vi "Apply Velocity to Wheels.vi"   [LabVIEW 2017, in "NI_Robotics_Steering Frame.lvclass"]
doc: "Calculates the state of each wheel necessary to satisfy the <B>steering frame velocity</B> or <B>arc velocity</B> at the center of the steering frame. You must manually select the polymorphic instance to use."
uses:
  <vilib>/robotics/Steering/Steering Frame/NI_Robotics_Steering Frame.lvclass
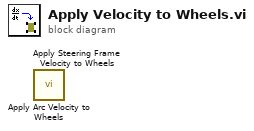
[diagram p0: block diagram]
diagram:
  n1 = call <vilib>:"Apply Arc Velocity to Wheels.vi"() -> ()  [unwired: 8 in, 4 out]
  n2 = call <vilib>:"Apply Steering Frame Velocity to Wheels.vi"() -> ()  [unwired: 8 in, 4 out]
